vi "Connect (SubVI).vi"(8 "error in (no error)":errorcluster, 11 "paramUnicornIn":T1) -> (0 "error out":errorcluster, 3 "paramUnicornIn out":T1)   [LabVIEW 2017, in "LV_Unicorn.lvlib"]
uses:
  LV_Unicorn.lvlib
  Control/unicorn_Param.ctl
  Control/unicorn_conn.ctl
  Control/unicorn_JSON.ctl
  Control/unicorn_ParamInt.ctl
  Control/unicorn_Telemetry.ctl
  Control/unicorn_Table.ctl
  Control/unicorn_ParamFloat.ctl
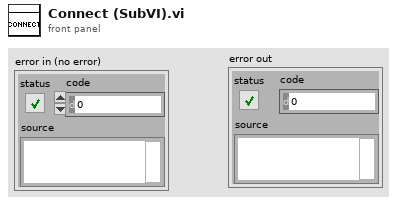
[diagram p1: front panel]
types:
  T1 = typedef "LV_Unicorn.lvlib/unicorn_Param.ctl" = cluster{"conParam":T2, "Param":T3}
  T2 = typedef "LV_Unicorn.lvlib/unicorn_conn.ctl" = cluster{"ReadIntParam":bool, "ReadDescrParam":bool, "ReadFloatParam":bool, "debug":bool, "ReadJSON":bool, "IP_address":string, "N_attempts":i32, "type_con":enum16{"Serial", "TCP"}, "MB_address":i32, "VISA":refnum<visa-resource-name>, "connection ID":refnum<k5>, "nameDevices":string, "timeout":i32, "port":u16, "type_version":string, "baud_rate":u32, "VersionControl":bool, "TCP_conn":bool, "WindowSize":i32}
  T3 = typedef "LV_Unicorn.lvlib/unicorn_JSON.ctl" = cluster{"NumParam":cluster{"NTelem":i32, "NInt":i32, "NFloat":i32, "NTable":i32}, "ParamInt":T4, "Telemetry":T5, "Table":T6, "ParamFloat":T7}
  T4 = typedef "LV_Unicorn.lvlib/unicorn_ParamInt.ctl" = cluster{"ID":string, "Num":i32, "Name":string, "Type":string, "Enum":string, "Desc":string, "Unit":string, "Access":string, "FormatStr":string, "Min":i32, "Max":i32}[]
  T5 = typedef "LV_Unicorn.lvlib/unicorn_Telemetry.ctl" = cluster{"ID":string, "Num":i32, "Name":string, "Desc":string, "Unit":string, "FormatStr":string, "Min":i32, "Max":i32}[]
  T6 = typedef "LV_Unicorn.lvlib/unicorn_Table.ctl" = cluster{"Num":i32, "Access":string, "ColumnCount":i32, "NeedParamPrepare":bool, "Columns":cluster{"Column":i32, "Desc":string, "Name":string}[], "DataType":string, "FormatStr":string, "ID":string, "Name":string, "RowCount":i32, "Rows":cluster{"Desc":string, "ID":string, "Max":i32, "Min":i32, "Name":string, "Row":i32, "Unit":string}[], "Type":string}[]
  T7 = typedef "LV_Unicorn.lvlib/unicorn_ParamFloat.ctl" = cluster{"ID":string, "Num":i32, "Name":string, "Type":string, "Enum":string, "Desc":string, "Unit":string, "Access":string, "FormatStr":string, "Min":sgl, "Max":sgl}[]
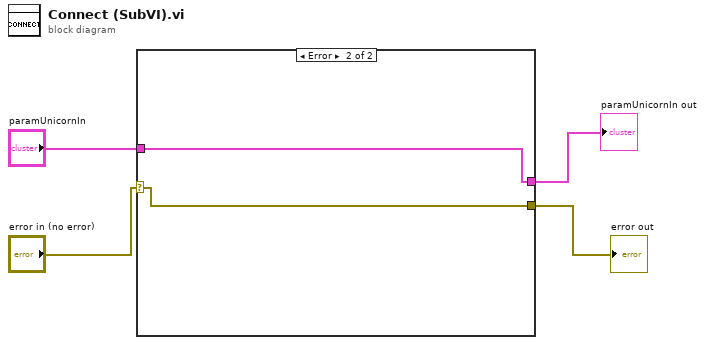
[diagram p0: block diagram]
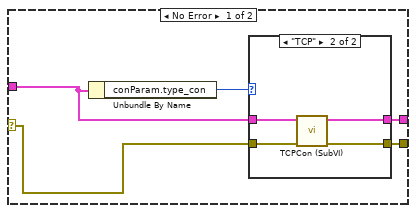
[diagram p2: hidden frame]
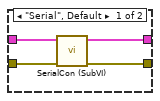
[diagram p3: hidden frame]
diagram:
  n1 = case shown="Error" "error in (no error)" {
    selector: "error in (no error)" -> [w5 w19]
    tunnel: [w9 w19] -> w4
    tunnel: [w8 w18] -> w3
    tunnel: "paramUnicornIn" -> [w7 w18]
    frame No Error {
      n2 = Unbundle By Name(w7) -> ("conParam.type_con"=w6:enum16{"Serial", "TCP"})
      n3 = case shown="\"TCP\"" w6 {
        tunnel: [w13 w17] -> w9
        tunnel: w5 -> [w10 w16]
        tunnel: w7 -> [w12 w15]
        tunnel: [w11 w14] -> w8
        frame "Serial", Default {
          n4 = call "SerialCon (SubVI).vi"("error in (no error)"=w10, "paramUnicornIn in"=w12) -> ("error out"=w13:errorcluster, "paramUnicornIn out"=w11:T1)  [unwired: 8 in]
        }
        frame "TCP" {
          n5 = call "TCPCon (SubVI).vi"("error in (no error)"=w16, "paramUnicornIn in"=w15) -> ("error out"=w17:errorcluster, "paramUnicornIn out"=w14:T1)  [unwired: 8 in]
        }
      }
    }
    frame Error {
    }
  }
  "error out" <- w4
  "paramUnicornIn out" <- w3
